vi "Move Back.vi"(8 "error in (no error)":errorcluster, 11 "Stage Controller in":refnum<class "Stage Controller.lvclass">) -> (0 "error out":errorcluster, 3 "Stage Controller out":refnum<class "Stage Controller.lvclass">)   [LabVIEW 2015, in "Stage Controller.lvlib" / "Stage Controller.lvclass"]
uses:
  Stage Controller.lvclass
  Stage Controller.lvclass/Stage Controller.ctl
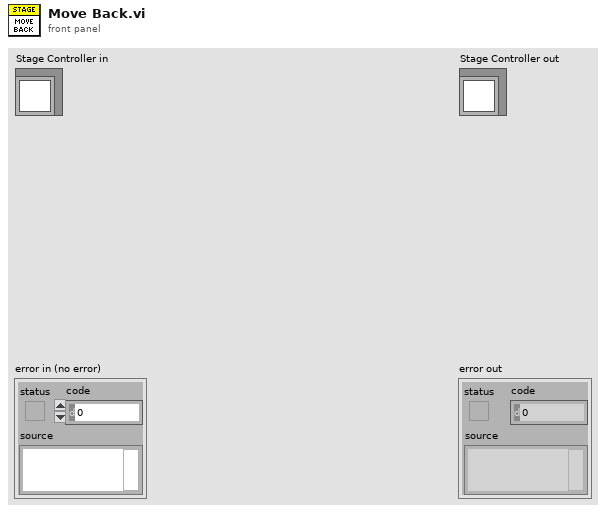
[diagram p1: front panel]
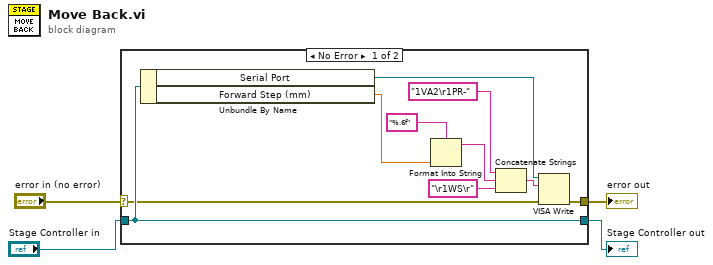
[diagram p0: block diagram]
diagram:
  n1 = case shown="No Error" "error in (no error)" {
    selector: "error in (no error)" -> [w6 w16]
    tunnel: [w5 w16] -> w3
    tunnel: [w14 w15] -> w1
    tunnel: "Stage Controller in" -> [w14 w15]
    frame No Error {
      n2 = Unbundle By Name(w14) -> ("Serial Port"=w13:refnum<visa-resource-name>, "Forward Step (mm)"=w10:dbl)
      n3 = Format Into String(format string="%.6f", w10) -> (resulting string=w8:string)  [unwired: 2 in, 1 out]
      n4 = Concatenate Strings("1VA2\r1PR-" ("write buffer"), w8, "\r1WS\r" ("write buffer")) -> (w7:string)
      n5 = VISA Write(VISA resource name=w13, write buffer=w7, error in (no error)=w6) -> (error out=w5:errorcluster)  [unwired: 2 out]
    }
    frame Error {
    }
  }
  "error out" <- w3
  "Stage Controller out" <- w1
